vi "MQTT_Read_Published_Message.vi"(8 "error in (no error)":errorcluster, 10 "timeout ms (25000)":i32=25000, 11 "connection ID":refnum<k5>) -> (0 "error out":errorcluster, 1 "Message":string="MQIsdp", 2 "Topic Name":string="Topic", 3 "connection ID out":refnum<k5>, 4 "MessageType":T1, 5 "Message ID":u16=1 format="%x")   [LabVIEW 2024, in "MQTT_Functions.lvlib"]
doc: "This VI reads the last published message at the selected topic. It sends acknowledge information if required by the QoS level.\n\n© 2015 - daq.io, LLC - Peter Adelhardt"
uses:
  MQTT_Functions.lvlib
  Controls/MessageType.ctl
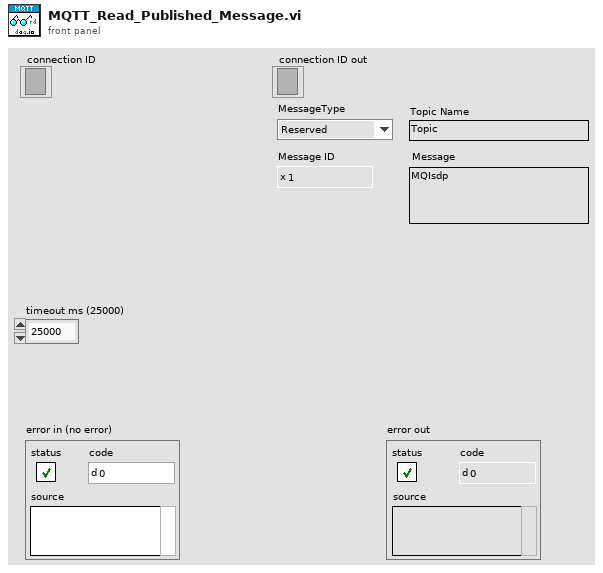
[diagram p1: front panel]
types:
  T1 = typedef "MQTT_Functions.lvlib/MessageType.ctl" = enum32{"Reserved", "CONNECT", "CONNACK", "PUBLISH", "PUBACK", "PUBREC", "PUBREL", "PUBCOMP", "SUBSCRIBE", "SUBACK", "UNSUBSCRIBE", "UNSUBACK", "PINGREQ", "PINGRESP", "DISCONNECT", "Reserved2"}
  T2 = typedef "MQTT_Functions.lvlib/QoS.ctl" = enum8{"At most once", "At least once", "Exactly once", "Reserved"}
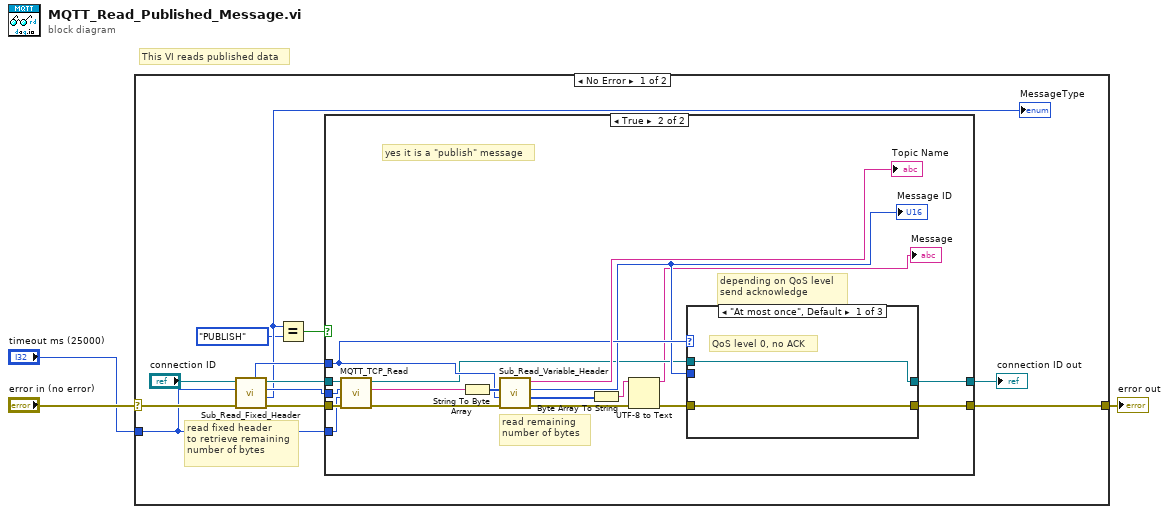
[diagram p0: block diagram]
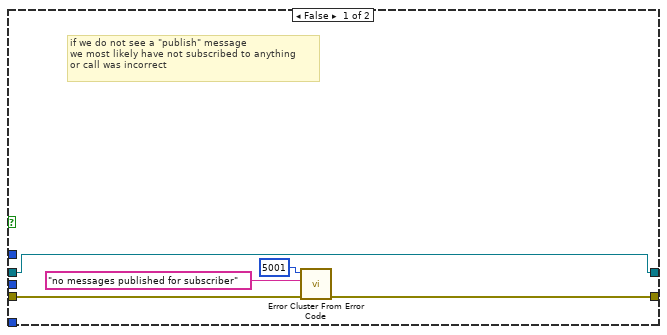
[diagram p2: hidden frame]
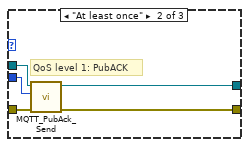
[diagram p3: hidden frame]
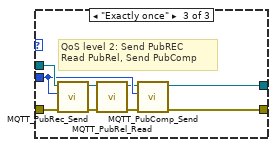
[diagram p4: hidden frame]
diagram:
  # "This VI reads published data"
  n1 = case shown="No Error" "error in (no error)" {
    selector: "error in (no error)" -> [w14 w55]
    tunnel: [w8 w55] -> w2
    tunnel: "timeout ms (25000)" -> [w4 _]
    frame No Error {
      # "read fixed header \nto retrieve remaining\nnumber of bytes"
      n2 = call "Sub_Read_Fixed_Header.vi"("error in (no error)"=w14, "timeout ms (25000)"=w4, "connection ID"="connection ID") -> ("error out"=w11:errorcluster, "MessageType"=w7:T1, "Remaining Length"=w13:u32, "connection ID out"=w12:refnum<k5>, "QoS Level"=w10:T2)  [unwired: 2 in, 2 out]
      "MessageType" <- w7
      n3 = Equal?(x=w7, y=MessageType."PUBLISH") -> (x = y?=w5:bool)
      n4 = case shown="True" w5 {
        tunnel: w13 -> [_ w37]
        tunnel: w12 -> [w16 w36]
        tunnel: w11 -> [w20 w35]
        tunnel: w10 -> [_ w31]
        tunnel: [w16 w28] -> w9
        tunnel: [w17 w27] -> w8
        tunnel: w4 -> [_ w21]
        frame False {
          # "if we do not see a \"publish\" message\nwe most likely have not subscribed to anything\nor call was incorrect"
          n5 = call <vilib>:"Error Cluster From Error Code.vi"("error in (no error)"=w20, "error message (\"\")"="no messages published for subscriber" ("error message (\"\")"), "error code (0)"=5001) -> ("error out"=w17:errorcluster)  [unwired: 6 in]
        }
        frame True {
          # "yes it is a \"publish\" message"
          # "depending on QoS level\nsend acknowledge"
          # "read remaining\nnumber of bytes"
          n6 = call "MQTT_TCP_Read.vi"("error in (no error)"=w35, "timeout ms (25000)"=w21, "bytes to read"=w37, "connection ID"=w36) -> ("error out"=w32:errorcluster, "data out"=w34:string, "connection ID out"=w29:refnum<k5>)  [unwired: 5 in]
          n7 = String To Byte Array(string=w34) -> (unsigned byte array=w33:u8[])
          n8 = call "Sub_Read_Variable_Header.vi"("error in (no error)"=w32, "QoS"=w31, "Variable Header"=w33) -> ("error out"=w22:errorcluster, "remaining bytes"=w26:u8[], "Message ID"=w30:u16, "Topic Name"=→"Topic Name":string)  [unwired: 5 in]
          "Message ID" <- w30
          n9 = Byte Array To String(unsigned byte array=w26) -> (string=w25:string)
          n10 = UTF-8 to Text(8:w22, 11:w25) -> (0:w23:errorcluster, 3:→"Message":string)  [unwired: 1 in]
          n11 = case shown="\"At most once\", Default" w31 {
            tunnel: w30 -> [_ w45 w50]
            tunnel: w23 -> [w39 w44 w54]
            tunnel: w29 -> [w40 w43 w53]
            tunnel: [w40 w42 w52] -> w28
            tunnel: [w39 w41 w51] -> w27
            frame "At most once", Default {
              # "QoS level 0, no ACK"
            }
            frame "At least once" {
              # "QoS level 1: PubACK"
              n12 = call "MQTT_PubAck_Send.vi"("error in (no error)"=w44, "Message ID"=w45, "connection ID"=w43) -> ("error out"=w41:errorcluster, "connection ID out"=w42:refnum<k5>)  [unwired: 6 in, 1 out]
            }
            frame "Exactly once" {
              # "QoS level 2: Send PubREC\nRead PubRel, Send PubComp"
              n13 = call "MQTT_PubRec_Send.vi"("error in (no error)"=w54, "Message ID"=w50, "connection ID"=w53) -> ("error out"=w47:errorcluster, "connection ID out"=w46:refnum<k5>)  [unwired: 6 in, 1 out]
              n14 = call "MQTT_PubRel_Read.vi"("error in (no error)"=w47, "connection ID"=w46) -> ("error out"=w48:errorcluster, "connection ID out"=w49:refnum<k5>)  [unwired: 7 in, 1 out]
              n15 = call "MQTT_PubComp_Send.vi"("error in (no error)"=w48, "Message ID"=w50, "connection ID"=w49) -> ("error out"=w51:errorcluster, "connection ID out"=w52:refnum<k5>)  [unwired: 6 in, 1 out]
            }
          }
        }
      }
      "connection ID out" <- w9
    }
    frame Error {
    }
  }
  "error out" <- w2
